vi "Parallel Mode Circuit Number of Second Secondary Channel Read Single.vi"(8 "error in":errorcluster, 9 "Channel Index":i32=1, 11 "Parallel Mode Channels In":refnum<class "Parallel Mode Channels.lvclass">) -> (0 "error out":errorcluster, 1 "Changed or First Call?":bool, 2 "Second Secondary Channel Circuit Number CTL":i32, 3 "Parallel Mode Channels Out":refnum<class "Parallel Mode Channels.lvclass">)   [LabVIEW 2023, in "Parallel Mode Channels.lvclass"]
uses:
  Parallel Mode Channels.lvclass
  Parallel Mode Channels.lvclass/Parallel Mode Channels.ctl
  <vilib>/ADAS Replay HIL/Channels/Tag Wrapper/Polymorphic/Read Channel (I32).vi
  a64bd9f8-41d0-4f13-b810-755f511eb55f.vi
  <vilib>/ADAS Replay HIL/Channels/Tag Wrapper/Polymorphic/Read Channel (I32).vi/b2f764de-0c1e-4784-a155-687fc995a684.vi
  <vilib>/ADAS Replay HIL/Channels/Tag Wrapper/Polymorphic/Read Channel (I32).vi/b2f764de-0c1e-4784-a155-687fc995a684.vi/c28b0ead-42ad-4072-80a2-aca7f2bd7ce3.vi
  <vilib>/ADAS Replay HIL/Channels/Tag Wrapper/Polymorphic/Read Channel (I32).vi/b2f764de-0c1e-4784-a155-687fc995a684.vi/219d0231-d98b-4193-b5cc-84f90e3c9091.vi
  <vilib>/ADAS Replay HIL/Channels/Tag Wrapper/Tag Wrapper.lvlib
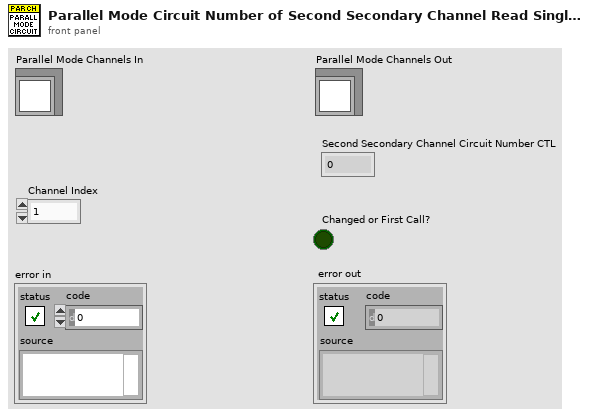
[diagram p1: front panel]
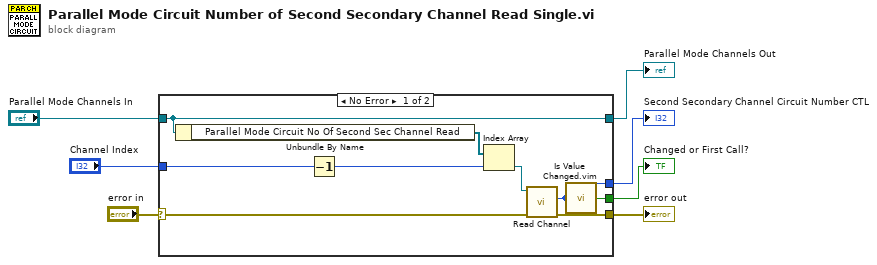
[diagram p0: block diagram]
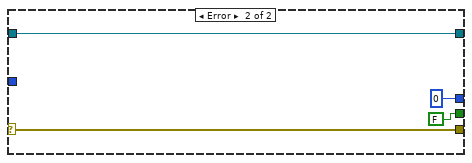
[diagram p2: hidden frame]
diagram:
  n1 = case shown="No Error" "error in" {
    selector: "error in" -> [w14 w20]
    tunnel: [w13 w20] -> w6
    tunnel: [w16 w19] -> w3
    tunnel: "Parallel Mode Channels In" -> [w16 w19]
    tunnel: [w12 0 ("Value out")] -> w1
    tunnel: [w11 FALSE ("changed or first call?")] -> w5
    tunnel: "Channel Index" -> [w10 _]
    frame No Error {
      n2 = Unbundle By Name(w16) -> ("Parallel Mode Circuit No Of Second Sec Channel Read"=w15:refnum<k21>[])
      n3 = Decrement(x=w10) -> (x-1=w9:i32)
      n4 = Index Array(array=w15, index=w9) -> (element=w8:refnum<k21>)
      n5 = call-poly <vilib>:"Read Channel.vi"("error in"=w14, "ADAS HIL Channel in"=w8) -> ("error out"=w13:errorcluster, "Value out"=w12:i32)  [unwired: 6 in, 2 out]
      n6 = call "Is Value Changed.vim"("value"=w12) -> ("changed or first call?"=w11:bool)
    }
    frame Error {
    }
  }
  "error out" <- w6
  "Changed or First Call?" <- w5
  "Parallel Mode Channels Out" <- w3
  "Second Secondary Channel Circuit Number CTL" <- w1
